vi "Read DAQmxTask dict.vi"(8 "error in (no error)":errorcluster, 11 "DAQmxTaskContainer_general in":refnum<class "DAQmxTaksContainer_General.lvclass">) -> (0 "error out":errorcluster, 2 "DAQmxTask dict":variant, 3 "DAQmxTaskContainer_general out":refnum<class "DAQmxTaksContainer_General.lvclass">)   [LabVIEW 2015, in "DAQmxTaksContainer_General.lvclass"]
uses:
  DAQmxTaksContainer_General.lvclass
  DAQmxTaksContainer_General.lvclass/DAQmxTaksContainer_General.ctl
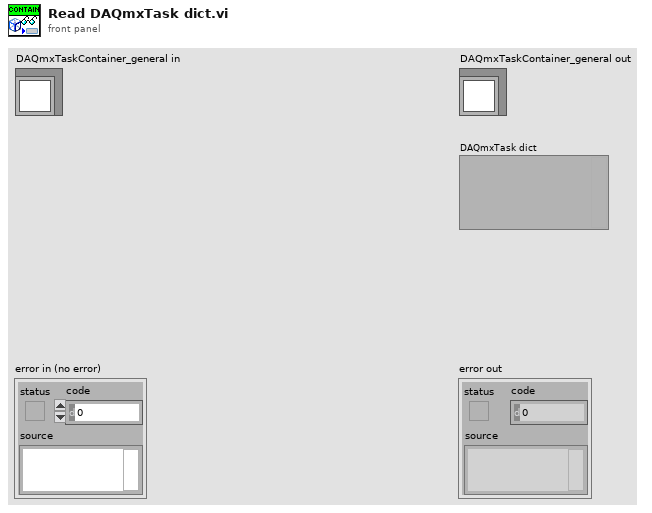
[diagram p1: front panel]
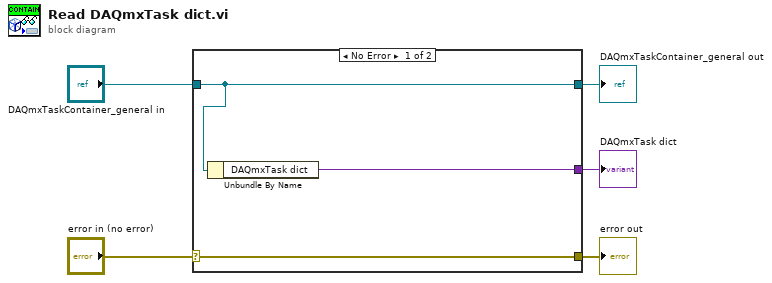
[diagram p0: block diagram]
diagram:
  n1 = case shown="No Error" "error in (no error)" {
    selector: "error in (no error)" -> [w8 w9]
    tunnel: [w8 w9] -> w4
    tunnel: [w6 w10] -> w2
    tunnel: "DAQmxTaskContainer_general in" -> [w6 w10]
    tunnel: [w7 _] -> w1
    frame No Error {
      n2 = Unbundle By Name(w6) -> ("DAQmxTask dict"=w7:variant)
    }
    frame Error {
    }
  }
  "error out" <- w4
  "DAQmxTaskContainer_general out" <- w2
  "DAQmxTask dict" <- w1
